vi "synch_mri_to_phys_data_v9.vi"() -> ()   [LabVIEW 2016]
uses:
  <vilib>/DAQmx/read.llb/DAQmx Read (Analog 1D DBL NChan 1Samp).vi
  <vilib>/DAQmx/create/channels.llb/DAQmx Create Channel (AI-Voltage-Basic).vi
  <vilib>/DAQmx/create/channels.llb/DAQmx Create Channel (DI-Digital Input).vi
  <vilib>/DAQmx/configure/timing.llb/DAQmx Timing (Sample Clock).vi
  <vilib>/Instr/_visa.llb/VISA Configure Serial Port (Instr).vi
  <vilib>/DAQmx/miscellaneous.llb/DAQmx Fill In Error Info.vi
  <vilib>/Utility/file.llb/Write Delimited Spreadsheet (DBL).vi
  <vilib>/Analysis/NI_AAL_SigProc.lvlib
  <vilib>/DAQmx/read.llb/DAQmx Read (Digital Bool 1Line 1Point).vi
panel:
  out "Pulse Value":dbl
  in  "pre-rec trig":dbl
  in  "Time":dbl
  in  "threshold":dbl=50.0 format="%#_13g"
  out "Trigger During Scan":dbl
  out "Time has elapsed":bool caption="Time has Elapsed"
  out "Elapsed Time (s)":dbl
  in  "Time Target (s)":dbl=600.0
  in  "Time recording?":bool=TRUE
  out "HR":dbl
  out "SpO2":dbl
  out "Temp":dbl
  out "Temp (deg C)":dbl(slide) scale=0.0..40.0
  out "% CO2":dbl format="%0.2f"
  in  "Dummy Count":dbl=8.0
  out "Trigger Pre-Scan":dbl
  in  "stop":bool
  out "trigger":cluster{"X":dbl[], "Y":dbl[]}[](graph) caption="XY Graph"
  in  "write file?":bool=TRUE
  out "Pulse":cluster{"Y":dbl[], "Y":dbl[]}[](graph)
  out "SpO_2":cluster{"Y":dbl[], "Y":dbl[]}[](graph)
  out "CO2":cluster{"Y":dbl[], "Y":dbl[]}[](graph)
  in  "file path (dialog if empty)":path
  in  "Test Run":bool
  out "read byte count":u32=15
  out "write byte count":u32=8
  in  "\"Get Temperature\" command":string="\u0006ùGVT\u0001ð>"
  in  "Sampling Rate":dbl=1000.0 format="%0.2f"
  in  "Mechanical Ventilator":tag="MRITrig/port0/line6"
  in  "CO2, SpO2, HR":tag="Dev0/ai2:4"
  in  "COM Port":refnum<visa-resource-name>="COM5"
  # "Trigger-sync Scan"
  # "Hardware Setup"
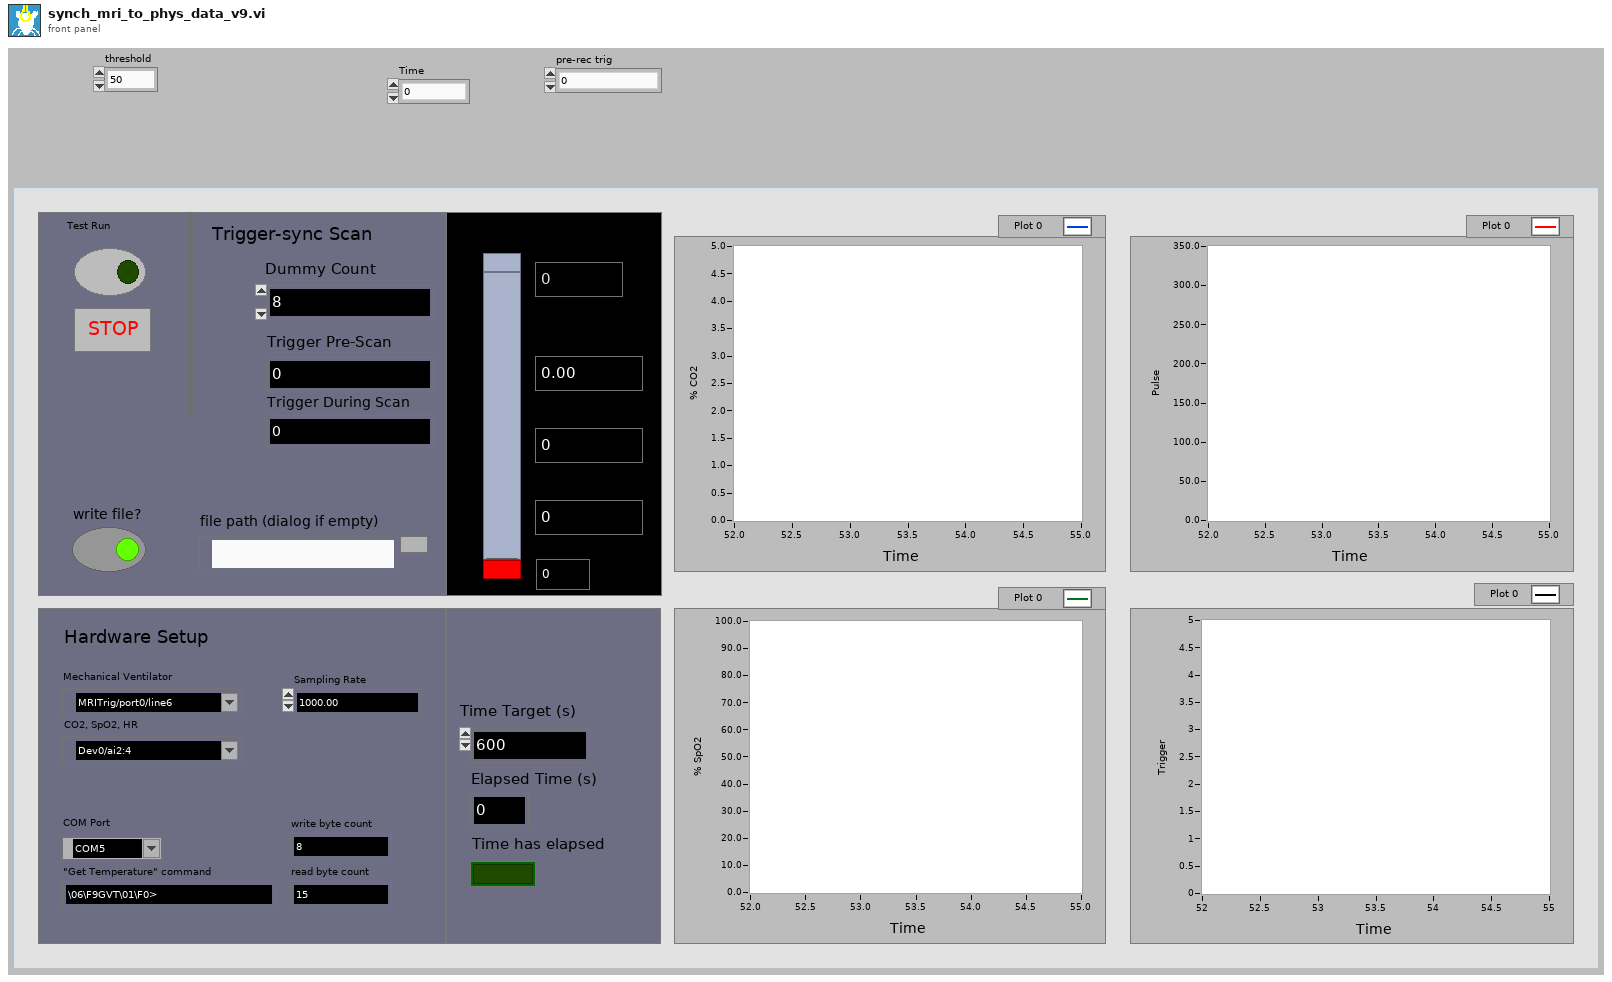
[diagram p1: front panel]
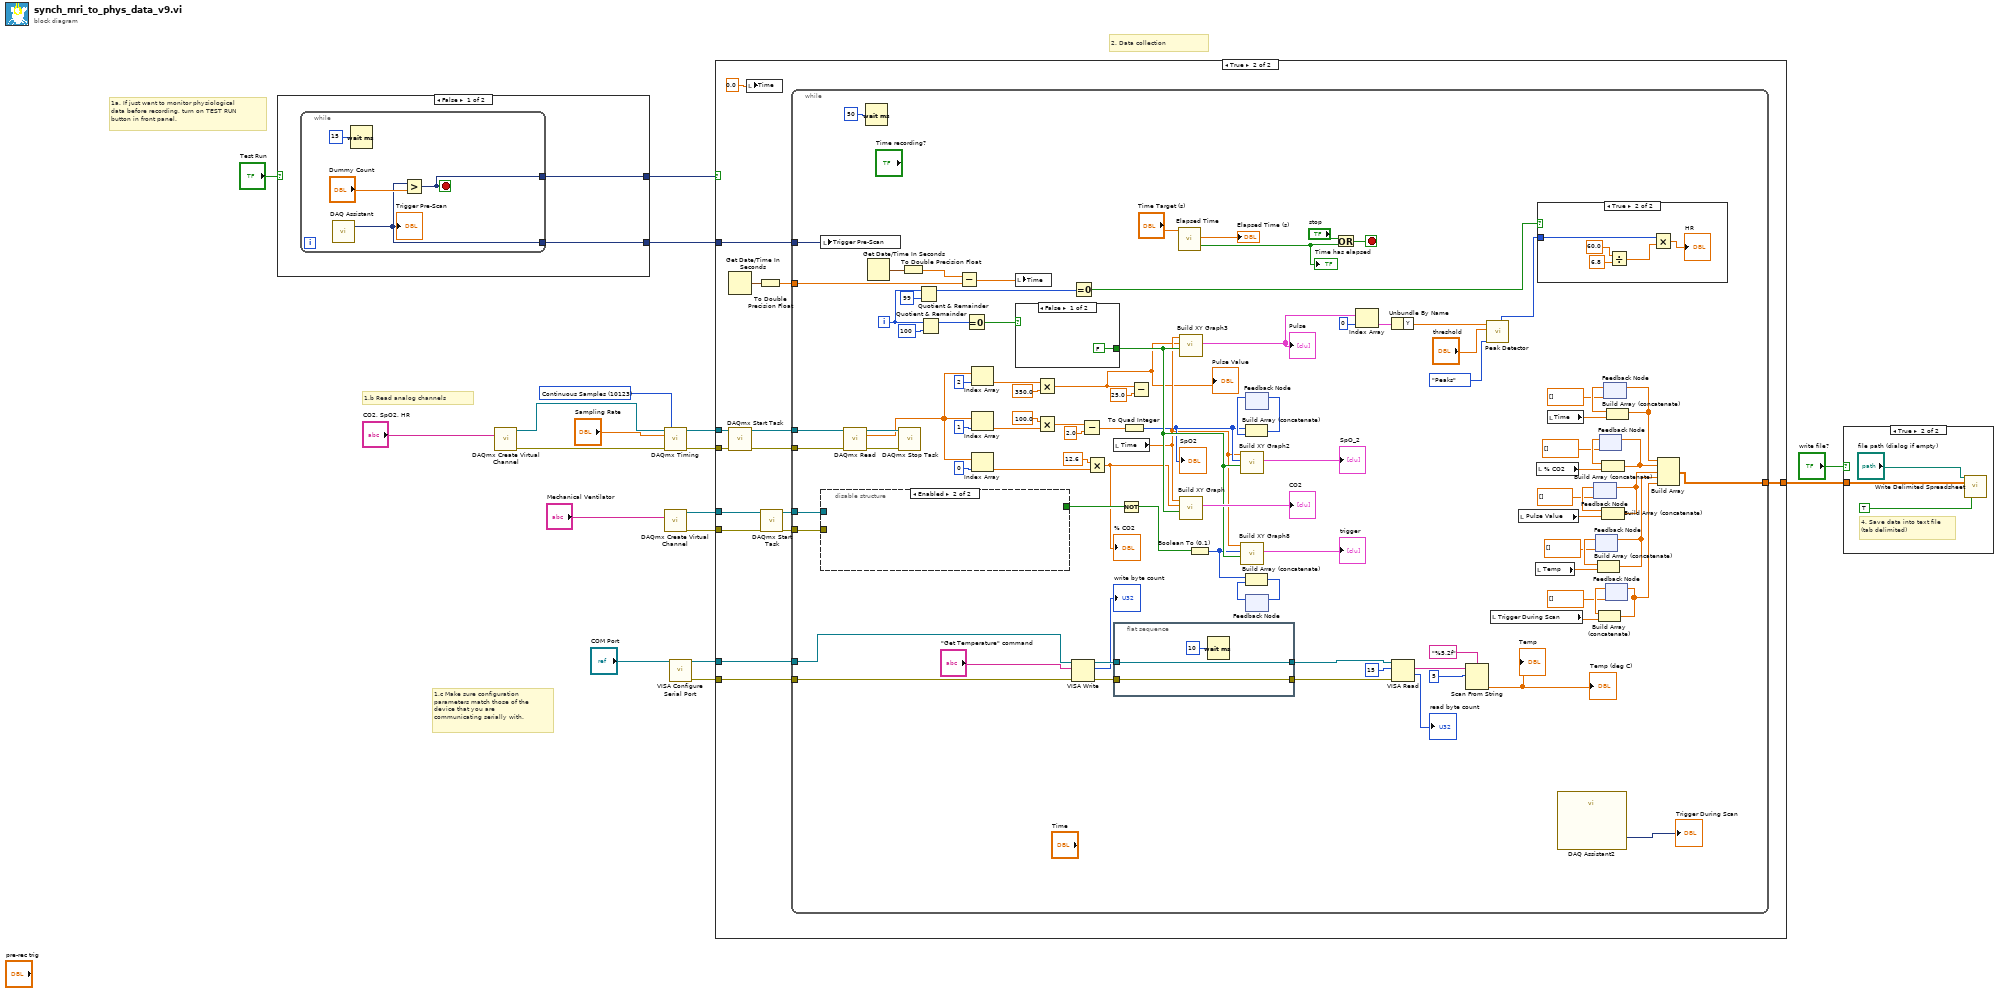
[diagram p0: block diagram]
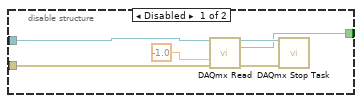
[diagram p5: hidden frame]
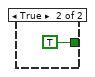
[diagram p6: hidden frame]
diagram:
  w14 = 10123 items=["Finite Samples"=10178, "Continuous Samples"=10123, "Hardware Timed Single Point"=12522] ("sample mode")
  # "2. Data collection"
  # "1.b Read analog channels"
  # "1a. If just want to monitor physiological\ndata before recording, turn on TEST RUN\nbutton in front panel."
  # "1.c Make sure configuration\nparameters match those of the \ndevice that you are \ncommunicating serially with."
  n1 = case shown="False" "Test Run" {
    selector: "Test Run" -> [_ w25]
    tunnel: [w20 _] -> w7
    tunnel: [w19 w25] -> w6
    frame False {
      n2 = while {
        tunnel: [w23] -> w20
        tunnel: [w22] -> w19
        stop <- w22 stop-if-true
        n3 = call "DAQ Assistant"() -> ("data"=w23:dynamicdata)  [unwired: 16 in, 3 out]
        "Trigger Pre-Scan" <- w23
        n4 = Wait (ms)(milliseconds to wait=u32 15) -> ()  [unwired: 1 out]
        n5 = Greater?(x=w23, y="Dummy Count") -> (0:w22:dynamicdata)
      }
    }
    frame True {
    }
  }
  n6 = call-poly <vilib>:"DAQmx Create Virtual Channel.vi"("physical channels"="CO2, SpO2, HR") -> ("task out"=w17:refnum<k21>, "error out"=w16:errorcluster)  [unwired: 13 in]
  n7 = call-poly <vilib>:"DAQmx Timing.vi"("task/channels in"=w17, "sample mode"=w14, "rate"="Sampling Rate", "error in"=w16) -> ("task out"=w2:refnum<k21>, "error out"=w1:errorcluster)  [unwired: 10 in]
  n8 = call-poly <vilib>:"DAQmx Create Virtual Channel.vi"("lines"="Mechanical Ventilator") -> ("task out"=w4:refnum<k21>, "error out"=w3:errorcluster)  [unwired: 13 in]
  n9 = call-poly "VISA Configure Serial Port"("VISA resource name"="COM Port") -> ("VISA resource name out"=w11:refnum<visa-resource-name>, "error out"=w10:errorcluster)  [unwired: 13 in]
  n10 = case shown="True" w6 {
    tunnel: w11 -> [_ w40]
    tunnel: w10 -> [_ w39]
    tunnel: [_ w38] -> w8
    tunnel: w7 -> [_ w37]
    tunnel: w4 -> [_ w32]
    tunnel: w3 -> [_ w31]
    tunnel: w2 -> [_ w30]
    tunnel: w1 -> [_ w29]
    frame False {
    }
    frame True {
      n11 = Get Date/Time In Seconds() -> (seconds since 1Jan1904=w27:timestamp)
      n12 = call <vilib>:"DAQmx Start Task.vi"("task/channels in"=w30, "error in"=w29) -> ("task out"=w34:refnum<k21>, "error out"=w35:errorcluster)  [unwired: 12 in]
      n13 = local write "Time"(0.0) -> ()
      n14 = To Double Precision Float(number=w27) -> (double precision float=w26:dbl)
      n15 = call <vilib>:"DAQmx Start Task.vi"("task/channels in"=w32, "error in"=w31) -> ("task out"=w36:refnum<k21>, "error out"=w33:errorcluster)  [unwired: 12 in]
      n16 = while {
        tunnel: w36 -> [w122]
        tunnel: w40 -> [w127]
        tunnel: w39 -> [w126]
        tunnel: [w121] -> w38
        tunnel: w37 -> [w89]
        tunnel: w35 -> [w63]
        tunnel: w34 -> [w64]
        tunnel: w33 -> [w62]
        tunnel: w26 -> [w59]
        i -> [w73]
        stop <- w114 stop-if-true
        n17 = local write "Trigger Pre-Scan"(w89) -> ()
        n18 = disable-structure shown="Enabled" {
          disable-tunnel: [w144 _] -> w94
          disable-tunnel: w122 -> [w143 _]
          disable-tunnel: w62 -> [w142 _]
          frame Disabled {
            n19 = call-poly <vilib>:"DAQmx Read.vi"("task/channels in"=w143, "timeout"=-1.0, "error in"=w142) -> ("task out"=w146:refnum<k21>, "data"=w144:bool, "error out"=w145:errorcluster)  [unwired: 10 in]
            n20 = call <vilib>:"DAQmx Stop Task.vi"("task/channels in"=w146, "error in"=w145) -> ()  [unwired: 12 in, 2 out]
          }
          frame Enabled {
          }
        }
        n21 = call-poly <vilib>:"DAQmx Read.vi"("task/channels in"=w64, "error in"=w63) -> ("task out"=w136:refnum<k21>, "data"=w117:dbl[], "error out"=w135:errorcluster)  [unwired: 11 in]
        n22 = Wait (ms)(milliseconds to wait=u32 50) -> ()  [unwired: 1 out]
        n23 = Get Date/Time In Seconds() -> (seconds since 1Jan1904=w61:timestamp)
        n24 = call <vilib>:"DAQmx Stop Task.vi"("task/channels in"=w136, "error in"=w135) -> ()  [unwired: 12 in, 2 out]
        n25 = To Double Precision Float(number=w61) -> (double precision float=w58:dbl)
        n26 = Quotient & Remainder(x=w73, y=99) -> (x-y*floor(x/y)=w81:i32)  [unwired: 1 out]
        n27 = Quotient & Remainder(x=w73, y=100) -> (x-y*floor(x/y)=w105:i32)  [unwired: 1 out]
        n28 = Subtract(x=w58, y=w59) -> (x-y=w57:dbl)
        n29 = Equal To 0?(x=w105) -> (x = 0?=w104:bool)
        n30 = Index Array(array=w117, index=2) -> (element=w95:dbl)
        n31 = Index Array(array=w117, index=1) -> (element=w107:dbl)
        n32 = Index Array(array=w117, index=0) -> (element=w109:dbl)
        n33 = local write "Time"(w57) -> ()
        n34 = case shown="False" w104 {
          tunnel: [FALSE ("Boolean 2") TRUE ("Boolean 2")] -> w103
          frame False {
          }
          frame True {
          }
        }
        n35 = Multiply(x=w95, y=350.0) -> (x*y=w56:dbl)
        "Pulse Value" <- w56
        n36 = Multiply(x=100.0, y=w107) -> (x*y=w90:dbl)
        n37 = VISA Write(VISA resource name=w127, write buffer="\"Get Temperature\" command", error in (no error)=w126) -> (VISA resource name out=w132:refnum<visa-resource-name>, return count=→"write byte count":u32, error out=w130:errorcluster)
        n38 = Equal To 0?(x=w81) -> (x = 0?=w80:bool)
        n39 = Subtract(x=w90, y=2.0) -> (x-y=w91:dbl)
        n40 = Multiply(x=12.6, y=w109) -> (x*y=w72:dbl)
        "% CO2" <- w72
        n41 = local read "Time"() -> (w66:dbl)
        n42 = flat-sequence {
          tunnel: [w152] -> w131
          tunnel: w132 -> [w152]
          tunnel: w130 -> [w151]
          tunnel: [w151] -> w129
          frame #0 {
            n43 = Wait (ms)(milliseconds to wait=u32 10) -> ()  [unwired: 1 out]
          }
        }
        n44 = Not(x=w94) -> (.not. x?=w93:bool)
        n45 = To Quad Integer(1:w91) -> (0:w96:i64)
        "SpO2" <- w96
        n46 = Subtract(x=w56, y=25.0) -> ()  [unwired: 1 out]
        n47 = call "Elapsed Time"("Time Target (s)"="Time Target (s)") -> ("Elapsed Time (s)"=→"Elapsed Time (s)":dbl, "Time has Elapsed"=w113:bool)  [unwired: 11 in, 6 out]
        "Time has elapsed" <- w113
        n48 = call "Build XY Graph3"("Reset"=w103, "Y Input"=w56, "X Input"=w66) -> ("XY Graph"=w87:cluster{"X":dbl[], "Y":dbl[]}[])  [unwired: 7 in, 1 out]
        "Pulse" <- w87
        n49 = call "Build XY Graph"("Reset"=w103, "Y Input"=w72, "X Input"=w66) -> ("XY Graph"=→"CO2":cluster{"X":dbl[], "Y":dbl[]}[])  [unwired: 7 in, 1 out]
        n50 = Boolean To (0,1)(Boolean=w93) -> (0, 1=w99:i16)
        n51 = call "Build XY Graph2"("Reset"=w103, "Y Input"=w96, "X Input"=w66) -> ("XY Graph"=→"SpO_2":cluster{"X":dbl[], "Y":dbl[]}[])  [unwired: 7 in, 1 out]
        n52 = call "Build XY Graph8"("Reset"=w103, "Y Input"=w99, "X Input"=w66) -> ("XY Graph"=→"trigger":cluster{"X":dbl[], "Y":dbl[]}[])  [unwired: 7 in, 1 out]
        n53 = feedback #1() -> (w102:i64[])  [unwired: 1 in]
        n54 = Build Array (concatenate)(w96, w102) -> (w101:i64[])
        n55 = feedback-in #1(w101) -> ()
        n56 = feedback #2() -> (w100:i16[])  [unwired: 1 in]
        n57 = Build Array (concatenate)(w99, w100) -> (w98:i16[])
        n58 = feedback-in #2(w98) -> ()
        n59 = Or(x="stop", y=w113) -> (x .or. y?=w114:bool)
        n60 = Index Array(array=w87, index=0) -> (element=w85:cluster{"X":dbl[], "Y":dbl[]})
        n61 = Unbundle By Name(w85) -> ("Y"=w78:dbl[])
        n62 = VISA Read(VISA resource name=w131, byte count=u32 15, error in (no error)=w129) -> (read buffer=w123:string, return count=→"read byte count":u32)  [unwired: 2 out]
        n63 = Scan From String(format string="%5.2f", input string=w123, initial scan location=u32 5) -> (output 1=→"Temp (deg C)" →"Temp":dbl)  [unwired: 2 in, 3 out]
        n64 = call <vilib>:"Peak Detector.vi"("peaks/valleys"=enum32{"Peaks", "Valleys"}."Peaks", "threshold"="threshold", "X"=w78) -> ("# found"=w79:i32)  [unwired: 4 in, 4 out]
        n65 = local read "Trigger During Scan"() -> (w53:dbl)
        n66 = local read "Pulse Value"() -> (w52:dbl)
        n67 = local read "Temp"() -> (w51:dbl)
        n68 = local read "% CO2"() -> (w50:dbl)
        n69 = case shown="True" w80 {
          tunnel: w79 -> [_ w138]
          frame False {
          }
          frame True {
            n70 = Divide(x=60.0, y=6.8) -> (x/y=w139:dbl)
            n71 = Multiply(x=w138, y=w139) -> (x*y=→"HR":dbl)
          }
        }
        n72 = local read "Time"() -> (w76:dbl)
        n73 = call "DAQ Assistant2"() -> ("data"=→"Trigger During Scan":dynamicdata)  [unwired: 16 in, 3 out]
        n74 = feedback #3(dbl[] []) -> (w70:dbl[])
        n75 = feedback #4(dbl[] []) -> (w68:dbl[])
        n76 = Build Array (concatenate)(w68, w51) -> (w67:dbl[])
        n77 = feedback-in #4(w67) -> ()
        n78 = feedback #5(dbl[] []) -> (w71:dbl[])
        n79 = Build Array (concatenate)(w71, w50) -> (w55:dbl[])
        n80 = feedback-in #5(w55) -> ()
        n81 = Build Array (concatenate)(w70, w52) -> (w69:dbl[])
        n82 = feedback-in #3(w69) -> ()
        n83 = feedback #6(dbl[] []) -> (w75:dbl[])
        n84 = feedback #7(dbl[] []) -> (w45:dbl[])
        n85 = Build Array (concatenate)(w45, w53) -> (w43:dbl[])
        n86 = feedback-in #7(w43) -> ()
        n87 = Build Array (concatenate)(w75, w76) -> (w54:dbl[])
        n88 = feedback-in #6(w54) -> ()
        n89 = Build Array(w54, w55, w69, w67, w43) -> (w121:dbl[][])
      }
    }
  }
  n90 = case shown="True" "write file?" {
    tunnel: w8 -> [_ w153]
    frame False {
    }
    frame True {
      # "4. Save data into text file \n(tab delimited)"
      n91 = call-poly <vilib>:"Write Delimited Spreadsheet.vi"("file path (dialog if empty)"="file path (dialog if empty)", "2D data"=w153, "transpose? (no:F)"=TRUE) -> ()  [unwired: 11 in, 2 out]
    }
  }
